vi "NTC拟合.vi"(11 "NTC电阻":dbl) -> (3 "NTC温度":dbl)   [LabVIEW 2021]
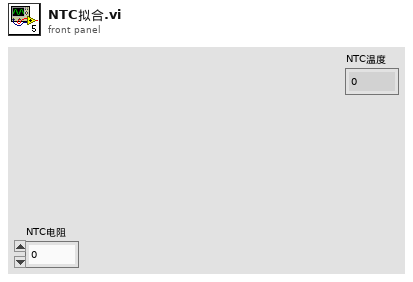
[diagram p1: front panel]
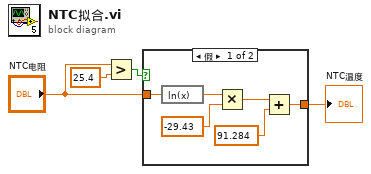
[diagram p0: block diagram]
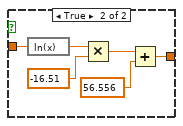
[diagram p2: hidden frame]
diagram:
  n1 = Greater?(x="NTC电阻", y=25.4) -> (0:w3:bool)
  n2 = case shown="假" w3 {
    tunnel: "NTC电阻" -> [w6 w16]
    tunnel: [w5 w11] -> w1
    frame False {
      n3 = expression code="ln(x)"(w6) -> (w9:dbl)
      n4 = Multiply(x=w9, y=-29.43) -> (x*y=w8:dbl)
      n5 = Add(x=w8, y=91.284) -> (x+y=w5:dbl)
    }
    frame True {
      n6 = expression code="ln(x)"(w16) -> (w14:dbl)
      n7 = Multiply(x=w14, y=-16.51) -> (x*y=w13:dbl)
      n8 = Add(x=w13, y=56.556) -> (x+y=w11:dbl)
    }
  }
  "NTC温度" <- w1
